vi "Assemble Coefficients.vi"(9 "Mtrx":dbl[][](array[numeric]), 10 "Triangle":i32[](array[numeric]), 11 "Sparse Matrix In":T1) -> (3 "Sparse Matrix Out":T1)   [LabVIEW 2020, in "Heat Equation Solver.lvlib"]
uses:
  Heat Equation Solver.lvlib
  <vilib>/Analysis/Matrix/Datatypes/RealMatrix.ctl
  <vilib>/Analysis/Matrix/NI_Matrix.lvlib
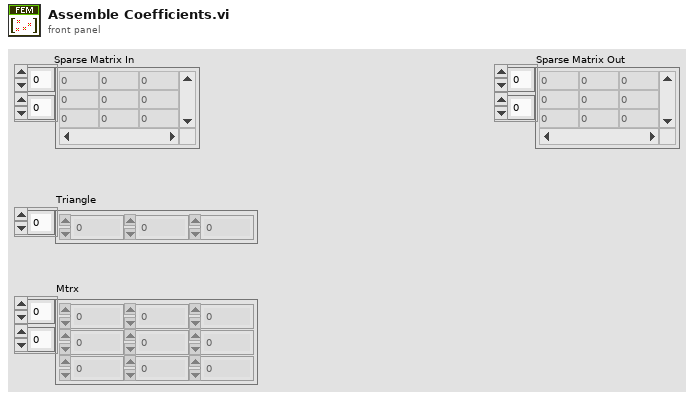
[diagram p1: front panel]
types:
  T1 = typedef "NI_Matrix.lvlib/RealMatrix.ctl" = dbl[][]
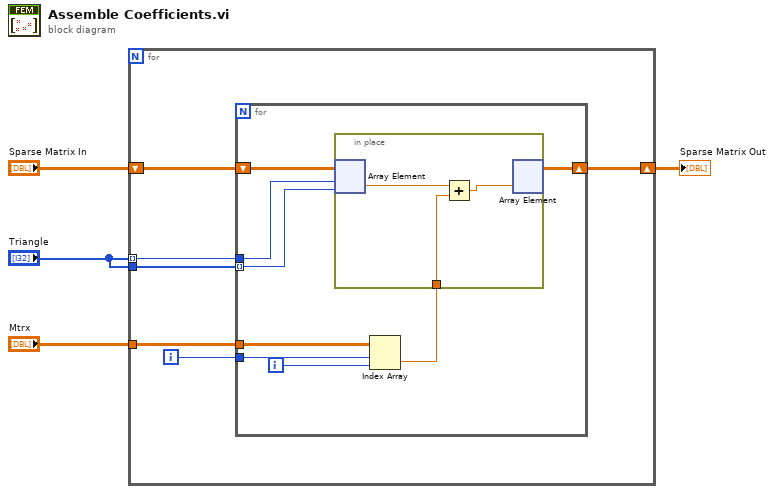
[diagram p0: block diagram]
diagram:
  n1 = for {
    tunnel: "Triangle" -> [w7] mode=indexing
    tunnel: "Triangle" -> [w10]
    tunnel: "Mtrx" -> [w9]
    shift-right: [w5] -> w2
    shift-left: "Sparse Matrix In" -> [w6]
    i -> [w8]
    n2 = for {
      tunnel: w10 -> [w13] mode=indexing
      tunnel: w7 -> [w14]
      tunnel: w9 -> [w18]
      tunnel: w8 -> [w17]
      shift-right: [w12] -> w5
      shift-left: w6 -> [w15]
      i -> [w16]
      n3 = Index Array(array=w18, index (row)=w17, index (col)=w16) -> (element=w11:dbl)
      n4 = in-place {
        in-place-border: w11 -> [w19]
        n5 = in-place-array #1(w15, w14, w13) -> (w21:dbl)
        n6 = Add(x=w21, y=w19) -> (x+y=w20:dbl)
        n7 = in-place-array #1(w20) -> (w12:T1)  [unwired: 2 out]
      }
    }
  }
  "Sparse Matrix Out" <- w2
